vi "Database.UpdateVariantFilesss.vi"(8 "error in (no error)":errorcluster, 11 "Data in":T1 {"Variant"."TS"."TV"."minimum" format="%#.3f"; "Variant"."TS"."TV"."maximum" format="%#.3f"; "Variant"."TS"."TP"."value" format="%#.3f"}) -> (0 "error out":errorcluster, 3 "Data out":T1 {"Variant"."TS"."TV"."minimum" format="%#.3f"; "Variant"."TS"."TV"."maximum" format="%#.3f"; "Variant"."TS"."TP"."value" format="%#.3f"})   [LabVIEW 2016]
uses:
  Database.Main.Data.ctl
  Database.Main.Data.Status.ctl
  Database.Main.Data.Sets.ctl
  Database.Main.Data.Results.ctl
  ProdaNG/Controls/ProdaNG.Identification.ctl
  ProdaNG/Controls/ProdaNG.ProcessResult.ctl
  ProdaNG/Controls/ProdaNG.ProcessStepResult.ctl
  ProdaNG/Controls/ProdaNG.TestStepResult.ctl
  ProdaNG/Controls/ProdaNG.TestValueResult.ctl
  Database.Main.Data.Variant.ctl
  ProdaNG/Controls/ProdaNG.ProcessStepParam.ctl
  ProdaNG/Controls/ProdaNG.TestStep.ctl
  ProdaNG/Controls/ProdaNG.TestStepParam.ctl
  ProdaNG/Controls/ProdaNG.TestValue.ctl
  Global/ApplicationGlobal.vi
panel:
  out "output 1":timestamp
  out "LatestChange":timestamp
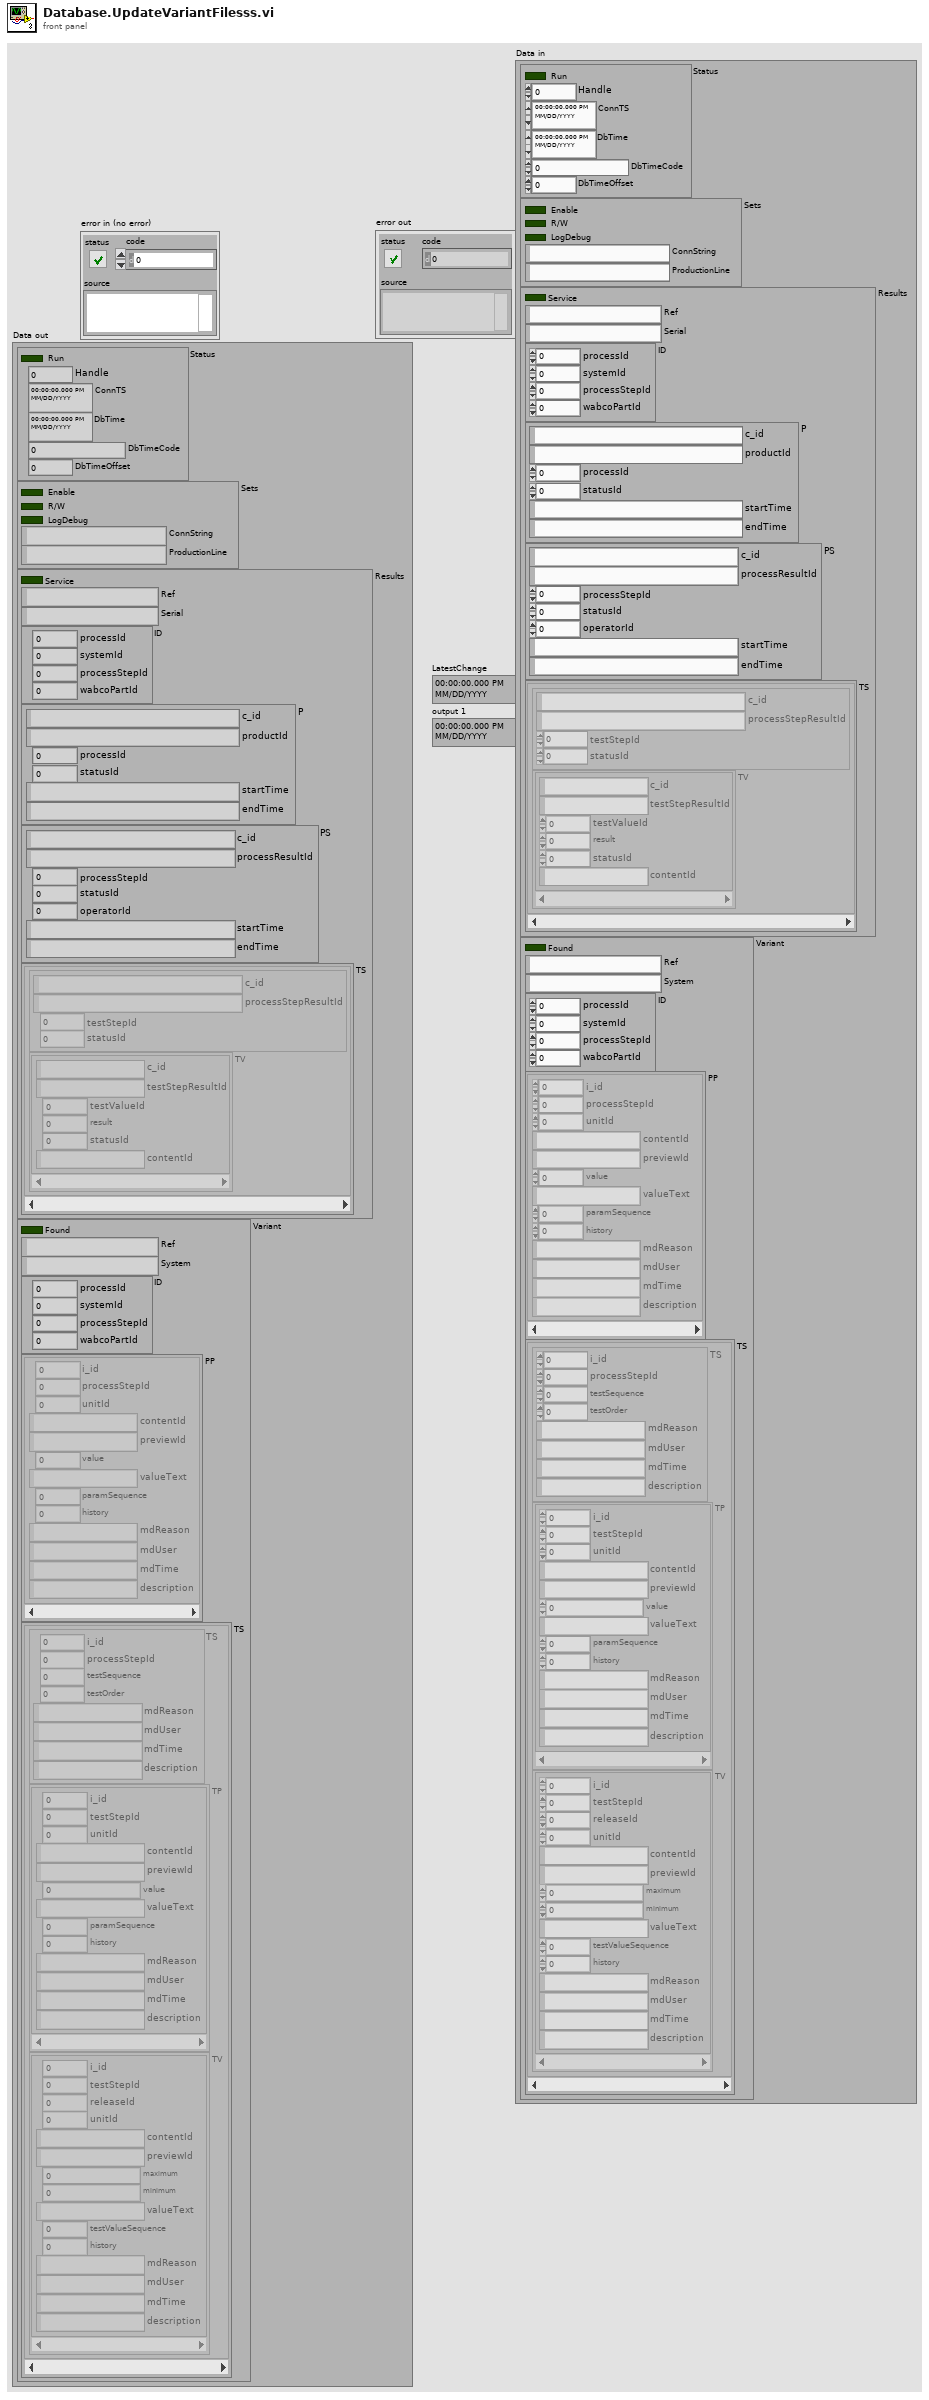
[diagram p1: front panel]
types:
  T1 = typedef "Database.Main.Data.ctl" = cluster{"Status":T2, "Sets":T3, "Results":T4, "Variant":T10}
  T2 = typedef "Database.Main.Data.Status.ctl" = cluster{"Run":bool, "Handle":i32, "ConnTS":timestamp, "DbTime":timestamp, "DbTimeCode":dbl, "DbTimeOffset":dbl}
  T3 = typedef "Database.Main.Data.Sets.ctl" = cluster{"Enable":bool, "R/W":bool, "LogDebug":bool, "ConnString":string, "ProductionLine":string}
  T4 = typedef "Database.Main.Data.Results.ctl" = cluster{"Service":bool, "Ref":string, "Serial":string, "ID":T5, "P":T6, "PS":T7, "TS":cluster{"TS":T8, "TV":T9[]}[]}
  T5 = typedef "ProdaNG.Identification.ctl" = cluster{"processId":i32, "systemId":i32, "processStepId":i32, "wabcoPartId":i32}
  T6 = typedef "ProdaNG.ProcessResult.ctl" = cluster{"c_id":string, "productId":string, "processId":i32, "statusId":i32, "startTime":string, "endTime":string}
  T7 = typedef "ProdaNG.ProcessStepResult.ctl" = cluster{"c_id":string, "processResultId":string, "processStepId":i32, "statusId":i32, "operatorId":i32, "startTime":string, "endTime":string}
  T8 = typedef "ProdaNG.TestStepResult.ctl" = cluster{"c_id":string, "processStepResultId":string, "testStepId":i32, "statusId":i32}
  T9 = typedef "ProdaNG.TestValueResult.ctl" = cluster{"c_id":string, "testStepResultId":string, "testValueId":i32, "result":dbl, "statusId":i32, "contentId":string}
  T10 = typedef "Database.Main.Data.Variant.ctl" = cluster{"Found":bool, "Ref":string, "System":string, "ID":T5, "PP":T11[], "TS":cluster{"TS":T12, "TP":T13[], "TV":T14[]}[]}
  T11 = typedef "ProdaNG.ProcessStepParam.ctl" = cluster{"i_id":i32, "processStepId":i32, "unitId":i32, "contentId":string, "previewId":string, "value":dbl, "valueText":string, "paramSequence":i32, "history":i32, "mdReason":string, "mdUser":string, "mdTime":string, "description":string}
  T12 = typedef "ProdaNG.TestStep.ctl" = cluster{"i_id":i32, "processStepId":i32, "testSequence":i32, "testOrder":i32, "mdReason":string, "mdUser":string, "mdTime":string, "description":string}
  T13 = typedef "ProdaNG.TestStepParam.ctl" = cluster{"i_id":i32, "testStepId":i32, "unitId":i32, "contentId":string, "previewId":string, "value":dbl, "valueText":string, "paramSequence":i32, "history":i32, "mdReason":string, "mdUser":string, "mdTime":string, "description":string}
  T14 = typedef "ProdaNG.TestValue.ctl" = cluster{"i_id":i32, "testStepId":i32, "releaseId":i32, "unitId":i32, "contentId":string, "previewId":string, "maximum":dbl, "minimum":dbl, "valueText":string, "testValueSequence":i32, "history":i32, "mdReason":string, "mdUser":string, "mdTime":string, "description":string}
  T15 = enum16{"open", "replace", "create", "open or create", "replace or create", "replace or create with confirmation"}
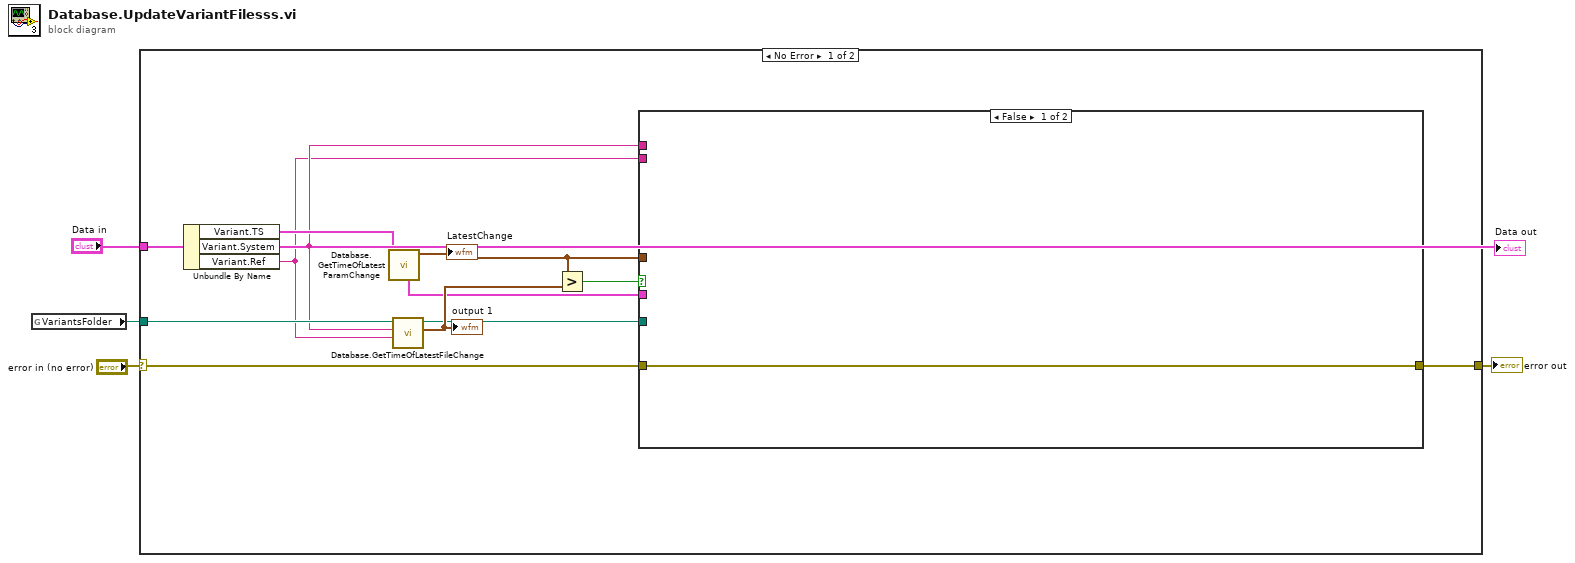
[diagram p0: block diagram]
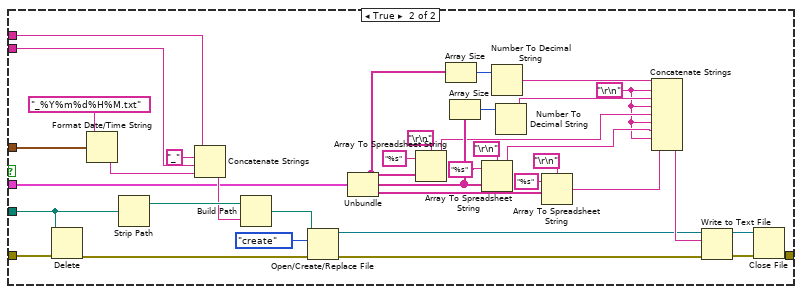
[diagram p2: hidden frame]
diagram:
  n1 = global read "ApplicationGlobal.vi" "VariantsFolder"() -> (w3:path)
  n2 = case shown="No Error" "error in (no error)" {
    selector: "error in (no error)" -> [w10 w55]
    tunnel: w3 -> [w14 _]
    tunnel: "Data in" -> [w16 _]
    tunnel: [w5 w55] -> w2
    frame No Error {
      n3 = Unbundle By Name(w16) -> ("Variant.TS"=w15:cluster{"TS":T12, "TP":T13[], "TV":T14[]}[], "Variant.System"=w8:string, "Variant.Ref"=w7:string)
      n4 = call "Database.GetTimeOfLatestParamChange.vi"("TS"=w15) -> ("Max"=w9:timestamp, "VariantFileValues"=w6:cluster{string[], string[], string[]})  [unwired: 6 in, 3 out]
      "LatestChange" <- w9
      n5 = call "Database.GetTimeOfLatestFileChange.vi"("Ref"=w7, "System"=w8, "VariantsFolder"=w14) -> ("Time Stamp"=w12:timestamp, "FilePath"=w11:path)  [unwired: 7 in]
      "output 1" <- w12
      n6 = Greater?(x=w9, y=w12) -> (0:w13:bool)
      n7 = case shown="False" w13 {
        tunnel: w11 -> [_ w51]
        tunnel: w10 -> [w17 w54]
        tunnel: w9 -> [_ w49]
        tunnel: w8 -> [_ w48]
        tunnel: w7 -> [_ w46]
        tunnel: w6 -> [_ w40]
        tunnel: [w17 w18] -> w5
        frame False {
        }
        frame True {
          w24 = "\r\n"
          n8 = Delete(path (use dialog)=w51, error in=w54) -> (error out=w53:errorcluster)  [unwired: 3 in, 2 out]
          n9 = Format Date/Time String(time format string (%c)="_%Y%m%d%H%M.txt" ("format string"), seconds (now)=w49) -> (date/time string=w45:string)  [unwired: 1 in]
          n10 = Strip Path(path=w51) -> (stripped path=w44:path)  [unwired: 1 out]
          n11 = Concatenate Strings(w48, "_" ("string"), w46, w45) -> (w43:string)
          n12 = Build Path(base path=w44, name or relative path=w43) -> (appended path=w42:path)
          n13 = Open/Create/Replace File(file path (use dialog)=w42, error in=w53, operation (0:open)=T15."create") -> (refnum out=w19:refnum<file>, error out=w41:errorcluster)  [unwired: 3 in, 1 out]
          n14 = Unbundle(w40) -> (w37:string[], w30:string[], w31:string[])
          n15 = Array To Spreadsheet String(delimiter (Tab)="\r\n", array=w37, 3:"%s" ("format string")) -> (spreadsheet string=w26:string)
          n16 = Array Size(array=w37) -> (size(s)=w36:i32)
          n17 = Array Size(array=w30) -> (size(s)=w29:i32)
          n18 = Array To Spreadsheet String(delimiter (Tab)="\r\n", array=w30, 3:"%s" ("format string")) -> (spreadsheet string=w25:string)
          n19 = Number To Decimal String(number=w36) -> (decimal integer string=w28:string)  [unwired: 1 in]
          n20 = Number To Decimal String(number=w29) -> (decimal integer string=w27:string)  [unwired: 1 in]
          n21 = Array To Spreadsheet String(delimiter (Tab)="\r\n", array=w31, 3:"%s" ("format string")) -> (spreadsheet string=w23:string)
          n22 = Concatenate Strings(w28, w24, w27, w24, w26, w24, w25, w24, w23) -> (w22:string)
          n23 = Write to Text File(file (use dialog)=w19, text=w22, error in=w41) -> (refnum out=w20:refnum<file>, error out=w21:errorcluster)  [unwired: 1 in, 1 out]
          n24 = Close File(refnum=w20, error in=w21) -> (error out=w18:errorcluster)  [unwired: 1 out]
        }
      }
    }
    frame Error {
    }
  }
  "error out" <- w2
  "Data out" <- "Data in"
